vi "Query Operation Status.vi"(8 "error in (no error)":errorcluster, 11 "VISA resource name":refnum<visa-resource-name>) -> (0 "error out":errorcluster, 1 "Acquire Status":u32(ring) items=["Busy"=0, "Acquire Idle"=1, "Wait For Acquire Trigger"=2, "Wait For Acquire Arm"=4], 2 "Transition Status":u32(ring) items=["Busy"=0, "Transition Idle"=1, "Wait For Transition Trigger"=2, "Wait For Transition Arm"=4], 3 "VISA resource name out":refnum<visa-resource-name>)   [LabVIEW 2012, in "Keysight B2980 Series.lvlib"]
doc: "Query the current instrument status."
uses:
  Keysight B2980 Series.lvlib
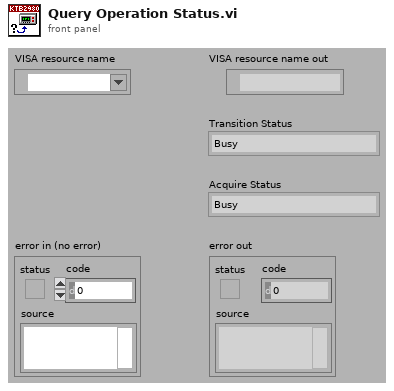
[diagram p1: front panel]
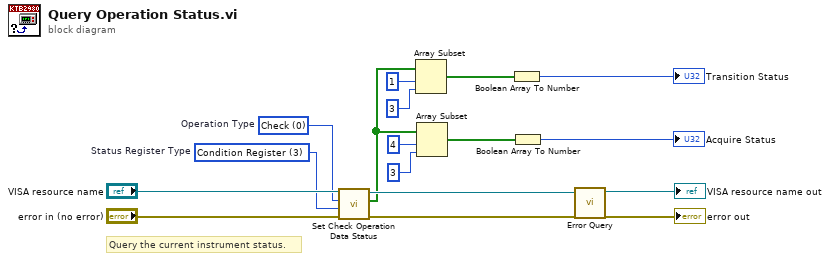
[diagram p0: block diagram]
diagram:
  w12 = 3 items=["Enable Register", "Negative Transition Filter Register", "Positive Transition Filter Register", "Condition Register", "Event Register"]  # Status Register Type
  w13 = 0 items=["Check", "Set"]  # Operation Type
  # "Query the current instrument status."
  n1 = call "Set Check Operation Data Status.vi"("error in (no error)"="error in (no error)", "Status Register Type (0: Enable Register)"=w12, "Operation Type (0: Check)"=w13, "VISA resource name"="VISA resource name") -> ("error out"=w10:errorcluster, "Register Status"=w2:bool[], "VISA resource name out"=w11:refnum<visa-resource-name>)  [unwired: 1 in, 4 out]
  n2 = Array Subset(array=w2, index=1, length=3) -> (w7:bool[])
  n3 = Array Subset(array=w2, index=4, length=3) -> (w3:bool[])
  n4 = Boolean Array To Number(Boolean array=w7) -> (number=→"Transition Status":u32)
  n5 = Boolean Array To Number(Boolean array=w3) -> (number=→"Acquire Status":u32)
  n6 = call "Error Query.vi"("error in (no error)"=w10, "VISA resource name"=w11) -> ("error out"=→"error out":errorcluster, "VISA resource name out"=→"VISA resource name out":refnum<visa-resource-name>)  [unwired: 8 out]
